vi "readRawFile.vi"() -> ()   [LabVIEW 2017]
panel:
  out "Error out":errorcluster
  in  "Raw File Path":path=path "F:/BonTechWrapperLibrary/BonTechWrapperLibrary/x64/Release/test.raw"
  in  "Length":i32=256
  in  "Frame Header":bool
  out "Image":T1(plugin-control)
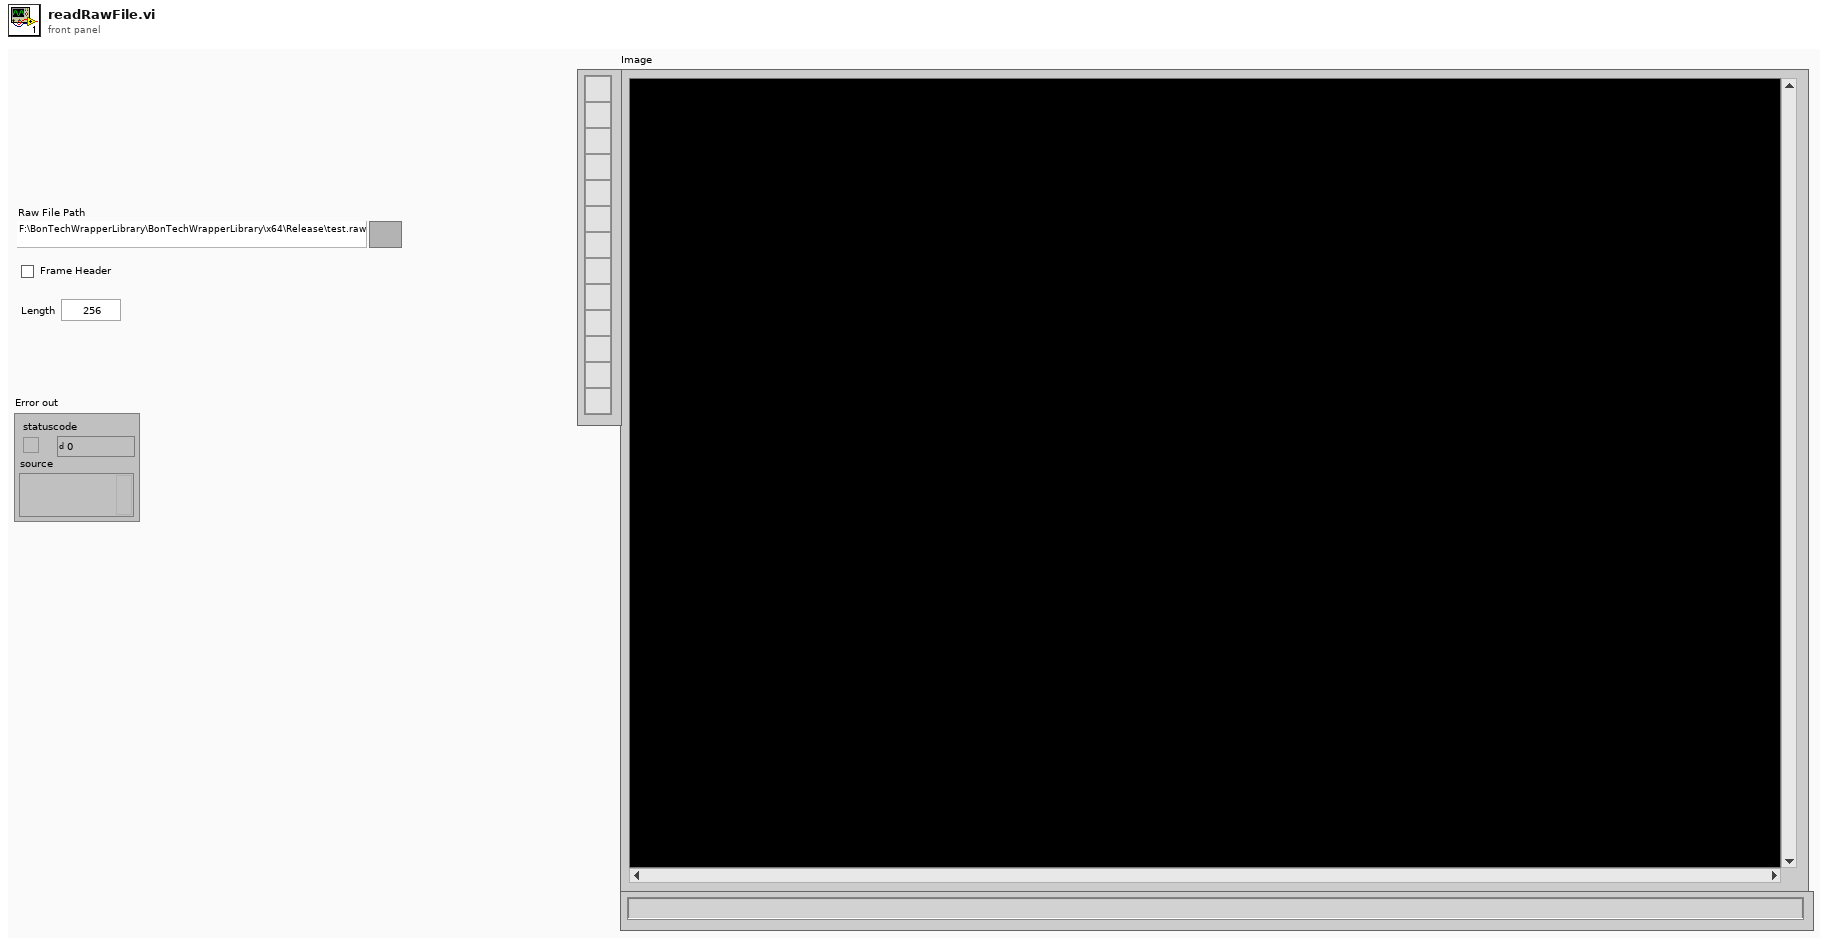
[diagram p1: front panel]
types:
  T1 = typedef "IMAQ Image.ctl" = refnum<image>
  T2 = typedef "Image Type" = u32
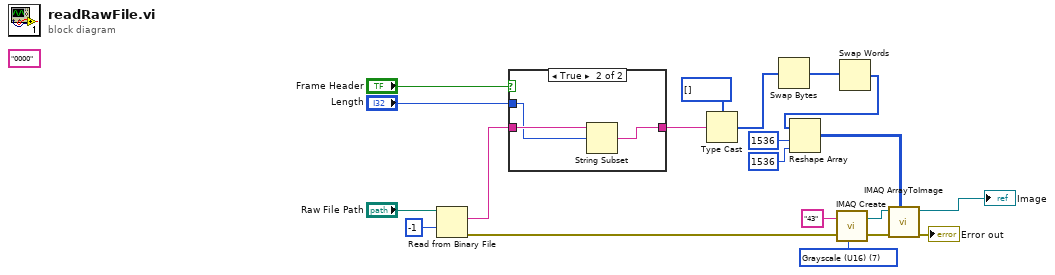
[diagram p0: block diagram]
diagram:
  w16 = T2 7 items=["Grayscale (U8)", "Grayscale (I16)", "Grayscale (SGL)", "Complex (CSG)", "RGB (U32)", "HSL (U32)", "RGB (U64)", "Grayscale (U16)"] ("Image Type")
  (unwired) "0000"
  n1 = Read from Binary File(10:-1 ("count (1)"), 11:"Raw File Path") -> (0:w5:errorcluster, 2:w8:string)  [unwired: 4 in, 2 out]
  n2 = case shown="True" "Frame Header" {
    tunnel: w8 -> [w21 w24]
    tunnel: "Length" -> [_ w22]
    tunnel: [w21 w23] -> w6
    frame False {
    }
    frame True {
      n3 = String Subset(string=w24, offset (0)=w22) -> (substring=w23:string)  [unwired: 1 in]
    }
  }
  n4 = Type Cast(type=u16[] [], x=w6) -> (*(type *) &x=w2:u16[])
  n5 = Swap Bytes(anything=w2) -> (byte swapped=w3:u16[])
  n6 = call "IMAQ Create"("Image Name"="43", "Image Type"=w16, "error in (no error)"=w5) -> ("New Image"=w15:T1, "error out"=w10:errorcluster)  [unwired: 2 in]
  n7 = Swap Words(1:w3) -> (0:w1:u16[])
  n8 = Reshape Array(w1, 1536 ("dimension size"), 1536 ("dimension size")) -> (w11:u16[][])
  n9 = call "IMAQ ArrayToImage"("Image Pixels (U16)"=w11, "error in (no error)"=w10, "Image"=w15) -> ("error out"=→"Error out":errorcluster, "Image Out"=→"Image":T1)  [unwired: 7 in]
